vi "SpareRelay_encode.vi"(8 "error in (no error)":errorcluster, 10 "Array":bool[](array[boolean])=[FALSE, FALSE, FALSE, FALSE, FALSE, FALSE, FALSE, FALSE, FALSE, FALSE, FALSE, FALSE, FALSE, FALSE, FALSE, FALSE, FALSE, FALSE, FALSE, FALSE], 11 "Mem_mapping in":u16[](array[numeric])) -> (0 "error out":errorcluster, 3 "MemMapping Out":u16[](array[numeric]))   [LabVIEW 2018, in "MB Relay.lvlib"]
uses:
  MB Relay.lvlib
panel:
  out "Data":u16[](array[numeric])
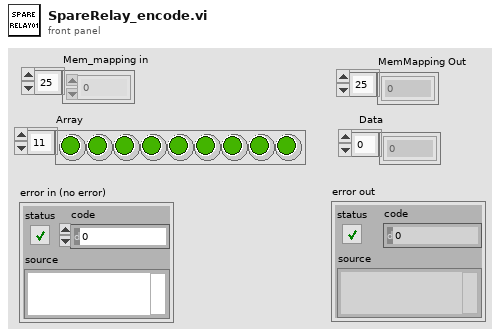
[diagram p1: front panel]
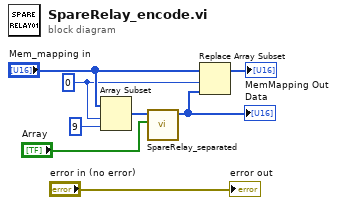
[diagram p0: block diagram]
diagram:
  w4 = 0 ("index")
  n1 = Array Subset(array="Mem_mapping in", index=w4, length=9) -> (w3:u16[])
  n2 = call "SpareRelay_separated.vi"("Array"="Array", "Mem_mapping in"=w3) -> ("Mem Mapping out"=w1:u16[])  [unwired: 9 in]
  "Data" <- w1
  n3 = Replace Array Subset(array="Mem_mapping in", new element=w1, index=w4) -> (→"MemMapping Out":u16[])
  "error out" <- "error in (no error)"
